vi "motor error handling.vi"(8 "error in (no error)":errorcluster, 11 "Handle in":i32) -> (0 "error out":errorcluster, 1 "Stop .vi?":bool, 2 "Handle Out out":i32, 3 "Error state":bool)   [LabVIEW 2013]
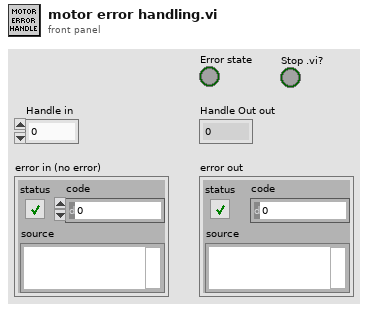
[diagram p1: front panel]
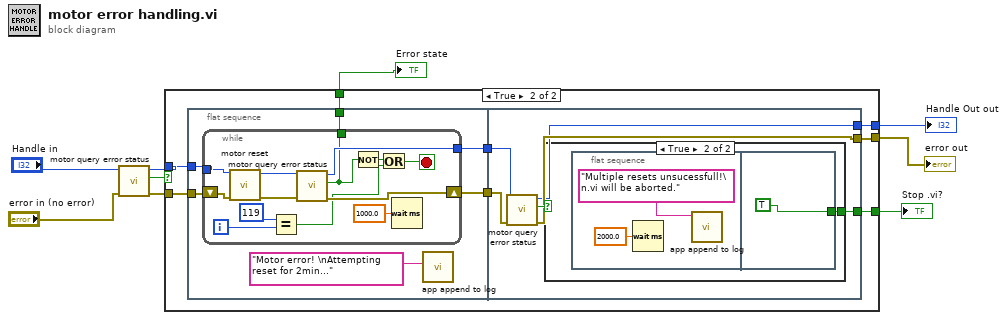
[diagram p0: block diagram]
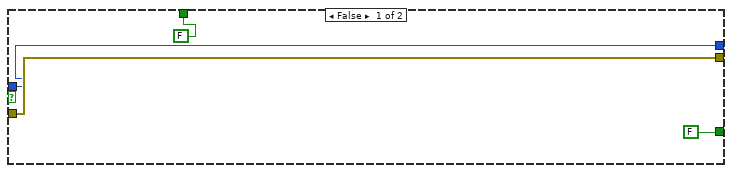
[diagram p2: hidden frame]
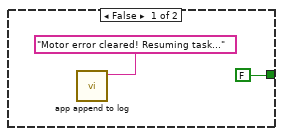
[diagram p3: hidden frame]
diagram:
  n1 = call "motor query error status.vi"("error in (no error)"="error in (no error)", "Handle In"="Handle in") -> ("error out"=w6:errorcluster, "Error state"=w4:bool, "Handle Out"=w5:i32)  [unwired: 7 in]
  n2 = case shown="True" w4 {
    tunnel: w5 -> [w12 w21]
    tunnel: w6 -> [w13 w20]
    tunnel: [w13 w18] -> w9
    tunnel: [w12 w16] -> w8
    tunnel: [FALSE w15] -> w2
    tunnel: [FALSE w14] -> w1
    frame False {
    }
    frame True {
      n3 = flat-sequence {
        tunnel: w21 -> [w27]
        tunnel: w20 -> [w25]
        tunnel: [w24] -> w19
        tunnel: [w23] -> w17
        tunnel: [w22] -> w15
        tunnel: w19 -> [w45]
        tunnel: [w44] -> w18
        tunnel: w17 -> [w43]
        tunnel: [w42] -> w16
        tunnel: [w41] -> w14
        frame #0 {
          n4 = while {
            tunnel: w27 -> [w39]
            shift-right: [w33] -> w24
            shift-left: w25 -> [w34]
            tunnel: [w32] -> w23
            tunnel: [w28] -> w22
            i -> [w36]
            stop <- w31 stop-if-true
            n5 = call "motor reset.vi"("error in (no error)"=w34, "Handle In"=w39) -> ("error out"=w37:errorcluster, "Handle Out"=w38:i32)  [unwired: 8 in]
            n6 = Equal?(x=119, y=w36) -> (x = y?=w29:bool)
            n7 = call "motor query error status.vi"("error in (no error)"=w37, "Handle In"=w38) -> ("error out"=w33:errorcluster, "Error state"=w28:bool, "Handle Out"=w32:i32)  [unwired: 7 in]
            n8 = Not(x=w28) -> (.not. x?=w30:bool)
            n9 = Or(x=w30, y=w29) -> (x .or. y?=w31:bool)
            n10 = Wait (ms)(milliseconds to wait=1000.0) -> ()  [unwired: 1 out]
          }
          n11 = call "app append to log.vi"("log line to append"="Motor error! \nAttempting reset for 2min...") -> ()  [unwired: 11 in]
        }
        frame #1 {
          n12 = call "motor query error status.vi"("error in (no error)"=w45, "Handle In"=w43) -> ("error out"=w44:errorcluster, "Error state"=w46:bool, "Handle Out"=w42:i32)  [unwired: 7 in]
          n13 = case shown="True" w46 {
            tunnel: [FALSE w49] -> w41
            frame False {
              n14 = call "app append to log.vi"("log line to append"="Motor error cleared! Resuming task...") -> ()  [unwired: 11 in]
            }
            frame True {
              n15 = flat-sequence {
                tunnel: [TRUE] -> w49
                frame #0 {
                  n16 = Wait (ms)(milliseconds to wait=2000.0) -> ()  [unwired: 1 out]
                  n17 = call "app append to log.vi"("log line to append"="Multiple resets unsucessfull!\n.vi will be aborted.") -> ()  [unwired: 11 in]
                }
                frame #1 {
                }
              }
            }
          }
        }
      }
    }
  }
  "error out" <- w9
  "Handle Out out" <- w8
  "Error state" <- w2
  "Stop .vi?" <- w1
